vi "关闭通信连接.vi"(8 "error in (no error)":errorcluster, 11 "串口通信类 in":refnum<class "串口通信类.lvclass">) -> (0 "error out":errorcluster, 3 "串口通信类 out":refnum<class "串口通信类.lvclass">)   [LabVIEW 2015, in "串口通信类.lvclass"]
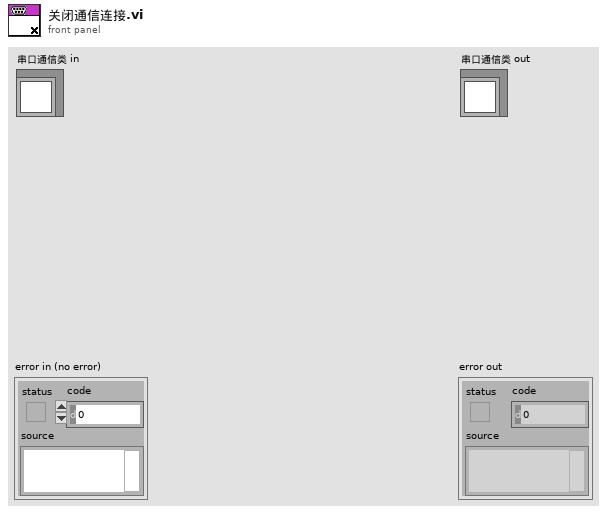
[diagram p1: front panel]
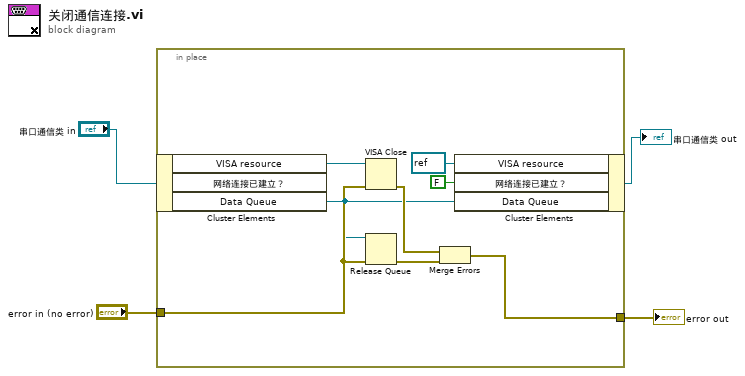
[diagram p0: block diagram]
diagram:
  n1 = in-place {
    in-place-border: "error in (no error)" -> [w9]
    in-place-border: [w6] -> w1
    n2 = in-place-cluster #1("串口通信类 in") -> ("VISA resource"=w12:refnum<visa-resource-name>, "Data Queue"=w5:refnum<queue>)  [unwired: 1 out]
    n3 = VISA Close(VISA resource name=w12, error in (no error)=w9) -> (error out=w8:errorcluster)
    n4 = Release Queue(queue=w5, error in (no error)=w9) -> (error out=w7:errorcluster)  [unwired: 1 in, 2 out]
    n5 = Merge Errors(w8, w7) -> (w6:errorcluster)
    n6 = in-place-cluster #1("VISA resource"=refnum<visa-resource-name> refnum, "网络连接已建立？"=FALSE ("通信状态.网络连接已建立？"), "Data Queue"=w5) -> (→"串口通信类 out":refnum<class "串口通信类.lvclass">)
  }
  "error out" <- w1
